vi "MDPtr Pack DoubleArr.vi"(7 "Copies Count(1)":i32=1, 9 "String Attribute":string, 10 "error in (no error)":errorcluster, 11 "Double Array":dbl[](array[numeric])) -> (2 "error out":errorcluster, 3 "HexStrPtr":T1)   [LabVIEW 2017, in "MDPtr.lvlib"]
uses:
  MDPtr.lvlib
  MDPtr TypeDef/MDPtr.ctl
  MDPtr TypeDef/MDPtr SupportedDataTypeDef.ctl
  MDPtr TypeDef/MDPtr DataFrame-DoubleArr.ctl
  MDPtr TypeDef/MDPtr DataFrame-Common.ctl
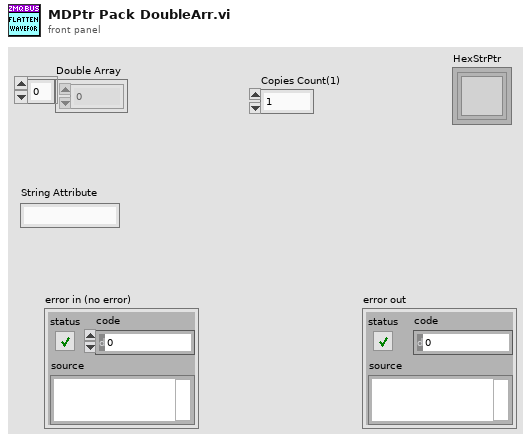
[diagram p1: front panel]
types:
  T1 = typedef "MDPtr.lvlib/MDPtr.ctl" = refnum<k1>
  T2 = typedef "MDPtr.lvlib/MDPtr DataFrame-DoubleArr.ctl" = cluster{"Common":T3, "DVR":refnum<data-value>}
  T3 = typedef "MDPtr.lvlib/MDPtr DataFrame-Common.ctl" = cluster{"Data Type":T4, "Copy Count":i32, "String Attribute":string}
  T4 = typedef "MDPtr.lvlib/MDPtr SupportedDataTypeDef.ctl" = enum16{"<Invalid>", "<User 0>", "<User 1>", "<User 2>", "<User 3>", "<User 4>", "Memory", "Waveform", "Waveform Arr", "Double Arr", "String Arr"}
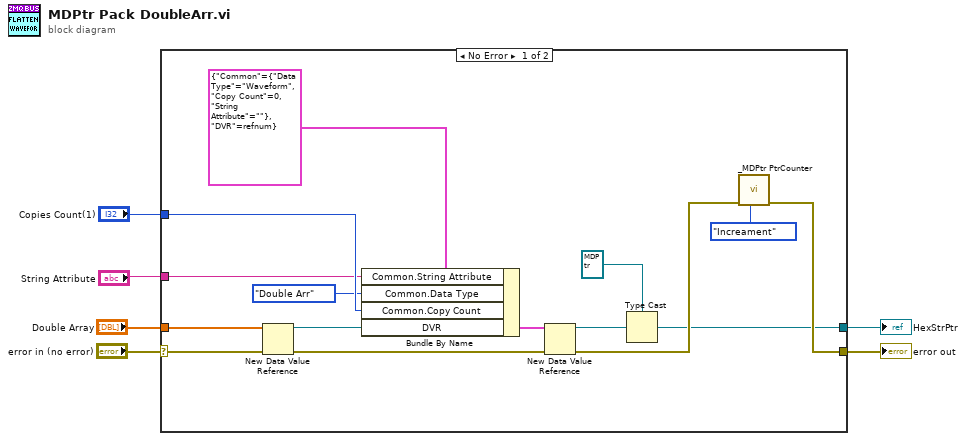
[diagram p0: block diagram]
diagram:
  n1 = case shown="No Error" "error in (no error)" {
    selector: "error in (no error)" -> [w20 w22]
    tunnel: [w16 w22] -> w5
    tunnel: "Double Array" -> [w14 _]
    tunnel: [w13 _] -> w3
    tunnel: "Copies Count(1)" -> [w11 _]
    tunnel: "String Attribute" -> [w7 _]
    frame No Error {
      n2 = New Data Value Reference(data value=w14, error in=w20) -> (data value reference=w12:refnum<data-value>, error out=w19:errorcluster)
      n3 = Bundle By Name(cluster=T2 {"Common"={"Data Type"=enum."Waveform", "Copy Count"=0, "String Attribute"=""}, "DVR"=refnum} ("DataFrame-Waveform Arr"), "Common.String Attribute"=w7, "Common.Data Type"=MDPtr_SupportedDataTypeDef."Double Arr" ("Data Type"), "Common.Copy Count"=w11, "DVR"=w12) -> (w21:T2)
      n4 = New Data Value Reference(data value=w21, error in=w19) -> (data value reference=w15:refnum<data-value>, error out=w17:errorcluster)
      n5 = Type Cast(type=T1 refnum ("MDPtr"), x=w15) -> (*(type *) &x=w13:T1)
      n6 = call "_MDPtr PtrCounter.vi"("Oper(Get)"=enum16{"GET", "Increament", "decreament"}."Increament", "error in (no error)"=w17) -> ("error out"=w16:errorcluster)  [unwired: 8 in, 1 out]
    }
    frame Error {
    }
  }
  "HexStrPtr" <- w3
  "error out" <- w5
